vi "Capture_Index.vi"(0 "Y":dbl=5.0, 5 "Amplitude (V)":dbl=5.0, 7 "Index_Select":T1) -> (4 "Capture?":bool)   [LabVIEW 2021]
doc: "This VI Captures the index points of transitions."
uses:
  Controls/Index_Select.ctl
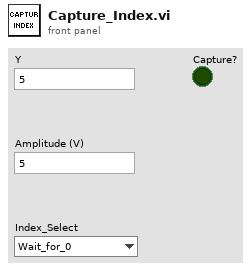
[diagram p1: front panel]
types:
  T1 = typedef "Index_Select.ctl" = enum16{"Wait_for_0", "Index_RTS", "Index_RTE", "Index_FTS", "Index_FTE"}
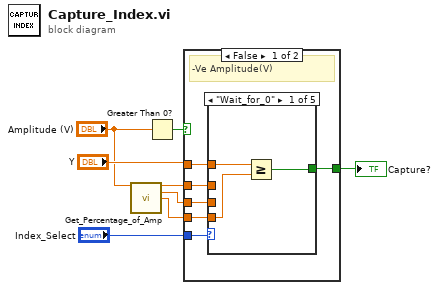
[diagram p0: block diagram]
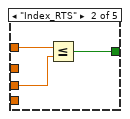
[diagram p2: hidden frame]
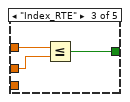
[diagram p3: hidden frame]
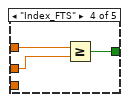
[diagram p4: hidden frame]
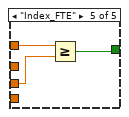
[diagram p5: hidden frame]
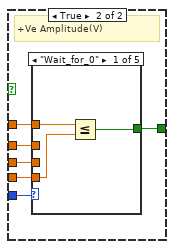
[diagram p6: hidden frame]
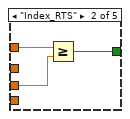
[diagram p7: hidden frame]
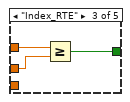
[diagram p8: hidden frame]
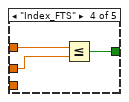
[diagram p9: hidden frame]
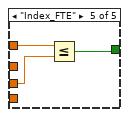
[diagram p10: hidden frame]
diagram:
  n1 = call "Get_Percentage_of_Amp.vi"("Amplitude(V)"="Amplitude (V)") -> ("End_Point"=w4:dbl, "Start_Point"=w3:dbl, "Min_Point"=w1:dbl)  [unwired: 12 in]
  n2 = Greater Than 0?(x="Amplitude (V)") -> (x > 0?=w7:bool)
  n3 = case shown="False" w7 {
    tunnel: "Index_Select" -> [w13 w35]
    tunnel: "Y" -> [w14 w34]
    tunnel: [w12 w33] -> w5
    tunnel: w4 -> [w11 w32]
    tunnel: w3 -> [w10 w31]
    tunnel: w1 -> [w9 w30]
    frame False {
      # "-Ve Amplitude(V)"
      n4 = case shown="\"Wait_for_0\"" w13 {
        tunnel: w14 -> [w17 w20 w23 w26 w29]
        tunnel: [w16 w19 w22 w25 w28] -> w12
        tunnel: w11 -> [_ _ w21 w24 _]
        tunnel: w9 -> [w15 _ _ _ _]
        tunnel: w10 -> [_ w18 _ _ w27]
        frame "Wait_for_0" {
          n5 = Greater Or Equal?(x=w17, y=w15) -> (x >= y?=w16:bool)
        }
        frame "Index_RTS" {
          n6 = Less Or Equal?(x=w20, y=w18) -> (x <= y?=w19:bool)
        }
        frame "Index_RTE" {
          n7 = Less Or Equal?(x=w23, y=w21) -> (x <= y?=w22:bool)
        }
        frame "Index_FTS" {
          n8 = Greater Or Equal?(x=w26, y=w24) -> (x >= y?=w25:bool)
        }
        frame "Index_FTE" {
          n9 = Greater Or Equal?(x=w29, y=w27) -> (x >= y?=w28:bool)
        }
      }
    }
    frame True {
      # "+Ve Amplitude(V)"
      n10 = case shown="\"Wait_for_0\"" w35 {
        tunnel: w34 -> [w38 w41 w44 w47 w50]
        tunnel: [w37 w40 w43 w46 w49] -> w33
        tunnel: w32 -> [_ _ w42 w45 _]
        tunnel: w30 -> [w36 _ _ _ _]
        tunnel: w31 -> [_ w39 _ _ w48]
        frame "Wait_for_0" {
          n11 = Less Or Equal?(x=w38, y=w36) -> (x <= y?=w37:bool)
        }
        frame "Index_RTS" {
          n12 = Greater Or Equal?(x=w41, y=w39) -> (x >= y?=w40:bool)
        }
        frame "Index_RTE" {
          n13 = Greater Or Equal?(x=w44, y=w42) -> (x >= y?=w43:bool)
        }
        frame "Index_FTS" {
          n14 = Less Or Equal?(x=w47, y=w45) -> (x <= y?=w46:bool)
        }
        frame "Index_FTE" {
          n15 = Less Or Equal?(x=w50, y=w48) -> (x <= y?=w49:bool)
        }
      }
    }
  }
  "Capture?" <- w5
